vi "Clusters.to.XML.vi"(8 "Mono":T2={"offset (cm-1)"=200.0, "step (cm-1)"=2.0, "Counter"=168.7592817604968, "Scanstep/monostep"=10, "Status"={"Moving"=FALSE, "Home"=FALSE, "Hi"=FALSE, "Low"=FALSE}, "nm"=675.0371270419872, "mono port"=""} {"nm" format="%.3f"; "Counter" format="%.2g"; "step (cm-1)" format="%.1f"}, 9 "DyeLaser":T3={"Scan.Start (cm-1)"=15000.0, "Scan.Stop (cm-1)"=15050.0, "Scan.step (cm-1)"=0.2, "dye laser port"="", "Laser"=enum."Syrah", "NSteps"=251, "CurrentStep"=75, "Current.cm-1"=15015.0} {"Current.cm-1" format="%.2f"}, 10 "Camera":T1={"Gate.Delay"=0, "Delay.Step"=0, "Gate.Duration"=150000, "#Accum"=10, "SetpointTemp"=-30, "Last Temp"=6, "Current Temp"=4}, 11 "XML File Path":path) -> ()   [LabVIEW 2022 SP3]
uses:
  <vilib>/Utility/xml.llb/Write to XML File(string).vi
panel:
  out "XML File Path out":path
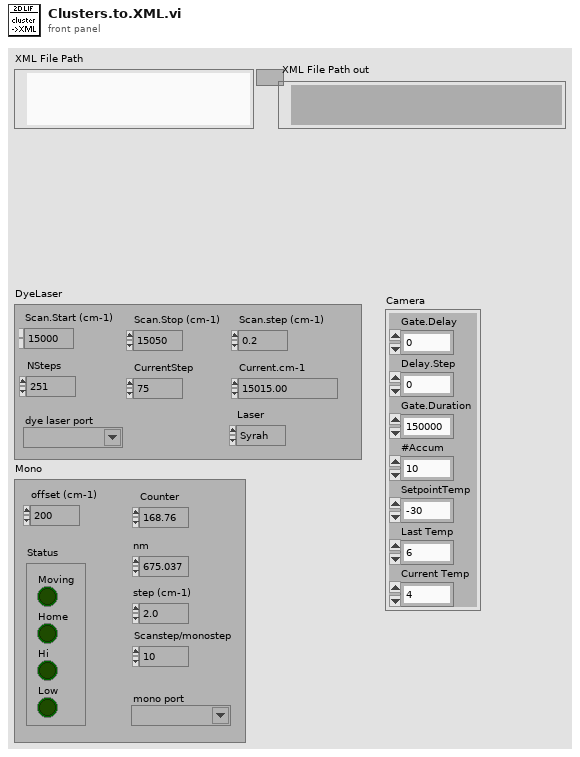
[diagram p1: front panel]
types:
  T1 = cluster{"Gate.Delay":u64, "Delay.Step":u64, "Gate.Duration":u64, "#Accum":i32, "SetpointTemp":i32, "Last Temp":i32, "Current Temp":i32}
  T2 = cluster{"offset (cm-1)":dbl, "step (cm-1)":dbl, "Counter":dbl, "Scanstep/monostep":i32, "Status":cluster{"Moving":bool, "Home":bool, "Hi":bool, "Low":bool}, "nm":dbl, "mono port":refnum<visa-resource-name>}
  T3 = cluster{"Scan.Start (cm-1)":dbl, "Scan.Stop (cm-1)":dbl, "Scan.step (cm-1)":dbl, "dye laser port":refnum<visa-resource-name>, "Laser":enum16{"Syrah", "Hyperdye"}, "NSteps":i32, "CurrentStep":i32, "Current.cm-1":dbl}
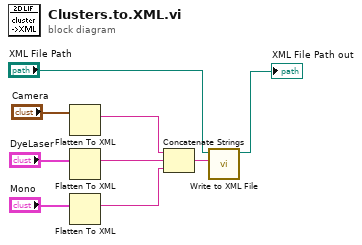
[diagram p0: block diagram]
diagram:
  n1 = Flatten To XML(6:"Camera") -> (2:w7:string)
  n2 = Flatten To XML(6:"DyeLaser") -> (2:w6:string)
  n3 = Flatten To XML(6:"Mono") -> (2:w5:string)
  n4 = Concatenate Strings(w7, w6, w5) -> (w4:string)
  n5 = call-poly <vilib>:"Write to XML File.vi"("XML Input"=w4, "XML File Path"="XML File Path") -> ("XML File Path(duplicate)"=→"XML File Path out":path)  [unwired: 7 in, 2 out]
